vi "Write Frame Data Recorder Multi Tool.vi"(8 "error in (no error)":errorcluster, 9 "Append":bool, 10 "Rigid Bodies":T1[](array[typedef]), 11 "Frame Grabber Data In in":T5={"Camera Session"="", "Frame"=refnum, "AVI Refnum"=refnum, "Codecs"=[], "Frame number"=0, "Tracking File Refnum"=refnum, "Tick Count"=0, "Probe Object"=refnum, "Playback Probe Data"=[], "Rigid Body"={"Position"={"x (mm)"=0.0, "y (mm)"=0.0, "z (mm)"=0.0}, "Orientation"={"Pitch (rad)"=0.0, "Yaw (rad)"=0.0, "Roll (rad)"=0.0}, "Quaternion"={"qx"=0.0, "qy"=0.0, "qz"=0.0, "qw"=0.0}, "Tracked?"=FALSE}, "Total no frames playback"=0, "Video FPS"=0.0, "Camera connected?"=FALSE, "Scene"=refnum, "Cropped Frame"=refnum, "Tracker FPS"=0.0, "Crop ROI"=[], "Presentation Values"=[], "Elapsed time (ms)"=0, "Camera frames playback"=0, "Refnums"={"Live Refnum"=refnum, "Record Refnum"=refnum, "Playback Refnum"=refnum, "Frame Slider Refnum"=refnum, "Pause Refnum"=refnum, "Home Refnum"=refnum, "Set Crop Refnum"=refnum, "Clear Crop Refnum"=refnum, "stop refnum"=refnum, "Playback Rate Refnum"=refnum, "Presentation Refnum"=refnum, "Crop Time Frame Slider Refnum"=refnum, "Cancel Save Refnum"=refnum, "Reverse Playback Refnum"=refnum, "Recording Settings Refnum"=refnum, "Continuous Playback Refnum"=refnum, "Annotation Refnum"=refnum, "Export All Refnum"=refnum, "Export List Refnum"=refnum, "Fill List Refnum"=refnum, "Save Crop Refnum"=refnum, "Skip Forward Refnum"=refnum, "Skip Backward Refnum"=refnum, "Single Annotation Refnum"=refnum, "Load Video Refnum"=refnum, "Set Start Refnum"=refnum, "Set End Refnum"=refnum, "Add to List Refnum"=refnum, "List of Annotations Refnum"=refnum, "Camera Frame Refnum"=refnum, "Load Image Refnum"=refnum, "Saving Refnum"=refnum}, "Dimensions"={"Probe Dimensions"={"Probe Width"=0.0, "Probe Depth"=1.0, "Probe Height"=0.0}, "Room Dimensions"={"Room Width"=0.0, "Room Depth"=0.0, "Room Height"=0.0}}, "Playback Data As Strings"=[], "Cropped Tracking File Refnum"=refnum, "Cropped AVI Refnum"=refnum, "Header"=[], "Total euclidian distance"=0.0, "Annotation File Path"=path "", "Playback File Path"=path "", "Size per frame"=0.0, "Ground Truth File Refnum"=refnum, "Annotation Array"=[], "Annotation TIFFs Folder"=path "", "overwriting open file?"=FALSE, "Image Sequence"=[], "Video/Image Flag"=enum."Playback Video Frame", "Image sequence?"=FALSE, "Image sequence filenames"=[], "Mask"=refnum, "Crop Type"=enum."Rectangle"}) -> (0 "error out":errorcluster, 1 "Time elapsed (s)":dbl, 2 "Image":T4, 3 "Frame Grabber Data out":T5={"Camera Session"="", "Frame"=refnum, "AVI Refnum"=refnum, "Codecs"=[], "Frame number"=0, "Tracking File Refnum"=refnum, "Tick Count"=0, "Probe Object"=refnum, "Playback Probe Data"=[], "Rigid Body"={"Position"={"x (mm)"=0.0, "y (mm)"=0.0, "z (mm)"=0.0}, "Orientation"={"Pitch (rad)"=0.0, "Yaw (rad)"=0.0, "Roll (rad)"=0.0}, "Quaternion"={"qx"=0.0, "qy"=0.0, "qz"=0.0, "qw"=0.0}, "Tracked?"=FALSE}, "Total no frames playback"=0, "Video FPS"=0.0, "Camera connected?"=FALSE, "Scene"=refnum, "Cropped Frame"=refnum, "Tracker FPS"=0.0, "Crop ROI"=[], "Presentation Values"=[], "Elapsed time (ms)"=0, "Camera frames playback"=0, "Refnums"={"Live Refnum"=refnum, "Record Refnum"=refnum, "Playback Refnum"=refnum, "Frame Slider Refnum"=refnum, "Pause Refnum"=refnum, "Home Refnum"=refnum, "Set Crop Refnum"=refnum, "Clear Crop Refnum"=refnum, "stop refnum"=refnum, "Playback Rate Refnum"=refnum, "Presentation Refnum"=refnum, "Crop Time Frame Slider Refnum"=refnum, "Cancel Save Refnum"=refnum, "Reverse Playback Refnum"=refnum, "Recording Settings Refnum"=refnum, "Continuous Playback Refnum"=refnum, "Annotation Refnum"=refnum, "Export All Refnum"=refnum, "Export List Refnum"=refnum, "Fill List Refnum"=refnum, "Save Crop Refnum"=refnum, "Skip Forward Refnum"=refnum, "Skip Backward Refnum"=refnum, "Single Annotation Refnum"=refnum, "Load Video Refnum"=refnum, "Set Start Refnum"=refnum, "Set End Refnum"=refnum, "Add to List Refnum"=refnum, "List of Annotations Refnum"=refnum, "Camera Frame Refnum"=refnum, "Load Image Refnum"=refnum, "Saving Refnum"=refnum}, "Dimensions"={"Probe Dimensions"={"Probe Width"=0.0, "Probe Depth"=1.0, "Probe Height"=0.0}, "Room Dimensions"={"Room Width"=0.0, "Room Depth"=0.0, "Room Height"=0.0}}, "Playback Data As Strings"=[], "Cropped Tracking File Refnum"=refnum, "Cropped AVI Refnum"=refnum, "Header"=[], "Total euclidian distance"=0.0, "Annotation File Path"=path "", "Playback File Path"=path "", "Size per frame"=0.0, "Ground Truth File Refnum"=refnum, "Annotation Array"=[], "Annotation TIFFs Folder"=path "", "overwriting open file?"=FALSE, "Image Sequence"=[], "Video/Image Flag"=enum."Playback Video Frame", "Image sequence?"=FALSE, "Image sequence filenames"=[], "Mask"=refnum, "Crop Type"=enum."Rectangle"}, 4 "File Size (MB)":dbl, 5 "Greater than 2 GB?":bool)   [LabVIEW 2017]
uses:
  Controls/Frame Grabber Data.ctl
  <vilib>/userdefined/High Color/IMAQdx.ctl
  <vilib>/vision/Image Controls.llb/IMAQ Image.ctl
  <vilib>/vision/Avi.llb/IMAQ AVI2 Refnum.ctl
  Controls/Rigid Body Info.ctl
  Controls/Position.ctl
  Controls/Orientation.ctl
  Controls/Refnums.ctl
  Controls/Recording Settings.ctl
  Controls/Operator Settings.ctl
  Controls/Operator.ctl
  Controls/Patient Settings.ctl
  Controls/Dimensions.ctl
  Controls/Room Dimensions.ctl
  Controls/Crop Video State.ctl
  Controls/Crop Type.ctl
panel:
  out "Camera frame number":dbl
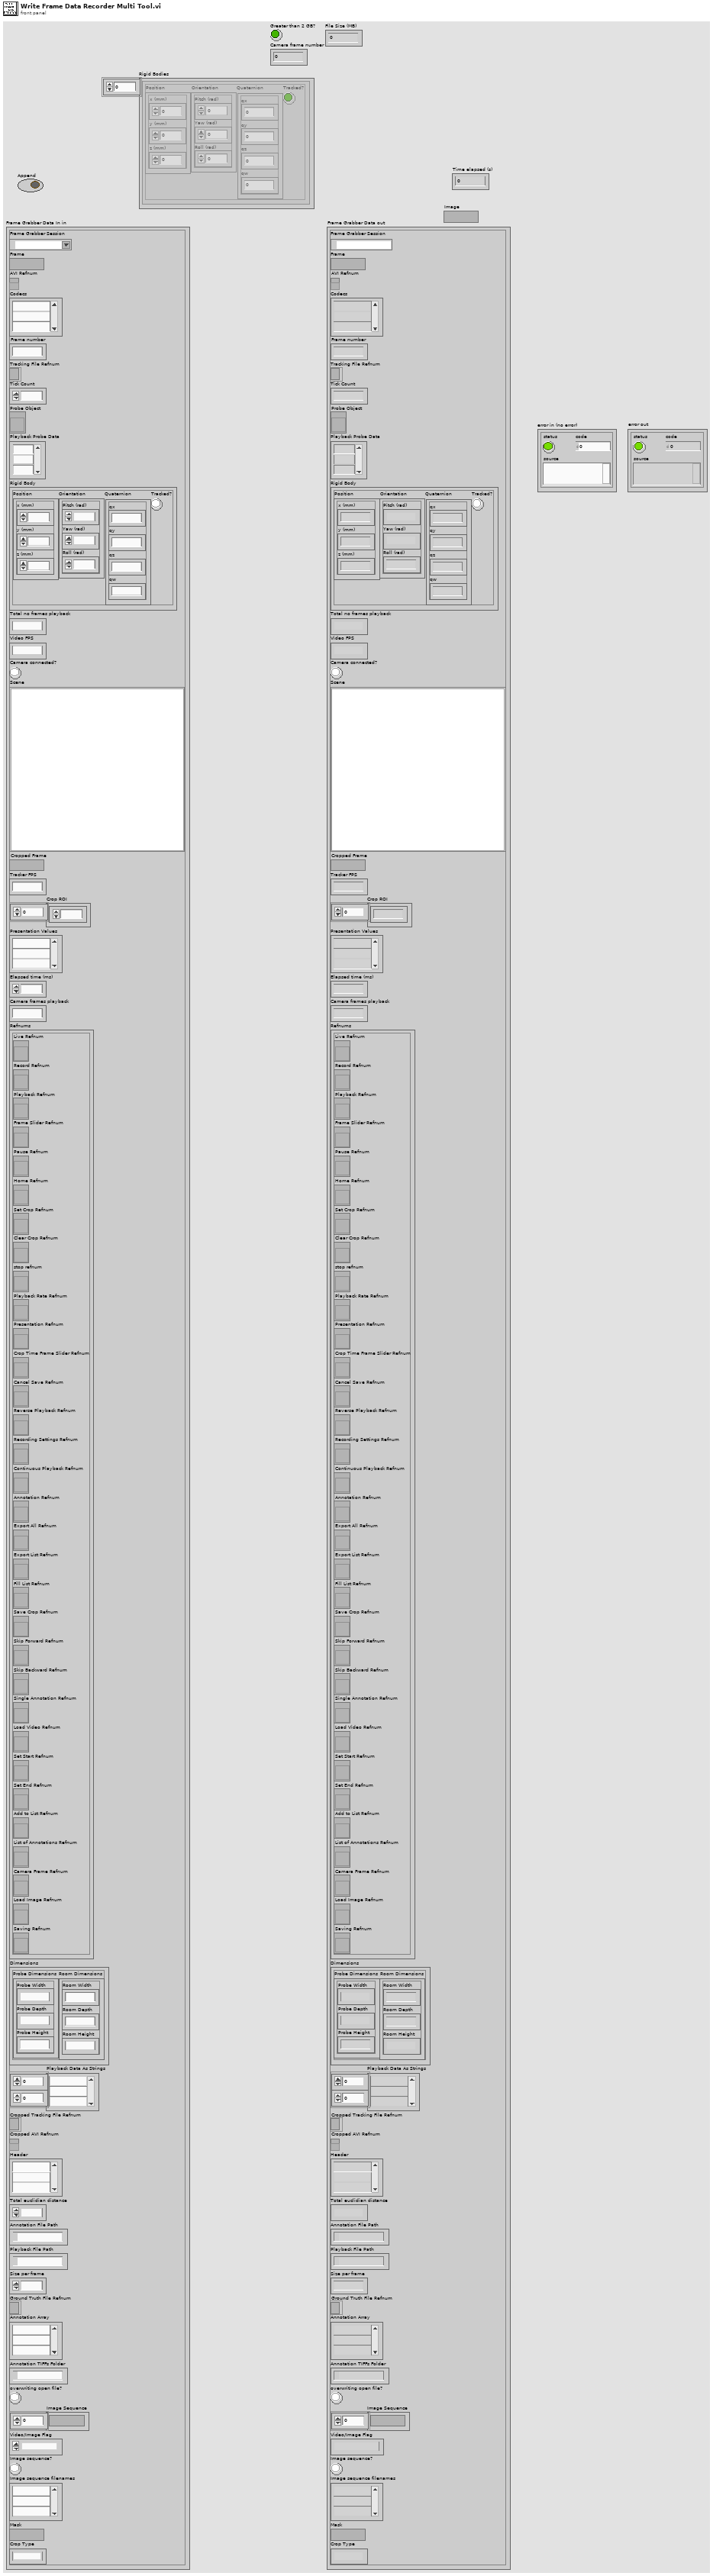
[diagram p1: front panel]
types:
  T1 = typedef "Rigid Body Info.ctl" = cluster{"Position":T2, "Orientation":T3, "Quaternion":cluster{"qx":sgl, "qy":sgl, "qz":sgl, "qw":sgl}, "Tracked?":bool}
  T2 = typedef "Position.ctl" = cluster{"x (mm)":sgl, "y (mm)":sgl, "z (mm)":sgl}
  T3 = typedef "Orientation.ctl" = cluster{"Pitch (rad)":sgl, "Yaw (rad)":sgl, "Roll (rad)":sgl}
  T4 = typedef "IMAQ Image.ctl" = refnum<image>
  T5 = typedef "Frame Grabber Data.ctl" = cluster{"Camera Session":T6, "Frame":T4, "AVI Refnum":T7, "Codecs":string[], "Frame number":u32, "Tracking File Refnum":refnum<file>, "Tick Count":u32, "Probe Object":refnum<vi>, "Playback Probe Data":dbl[][], "Rigid Body":T1, "Total no frames playback":i32, "Video FPS":dbl, "Camera connected?":bool, "Scene":refnum<vi>, "Cropped Frame":T4, "Tracker FPS":dbl, "Crop ROI":i32[], "Presentation Values":string[], "Elapsed time (ms)":u32, "Camera frames playback":u32, "Refnums":T8, "Dimensions":T9, "Playback Data As Strings":string[][], "Cropped Tracking File Refnum":refnum<file>, "Cropped AVI Refnum":T7, "Header":string[], "Total euclidian distance":dbl, "Annotation File Path":path, "Playback File Path":path, "Size per frame":dbl, "Ground Truth File Refnum":refnum<file>, "Annotation Array":string[], "Annotation TIFFs Folder":path, "overwriting open file?":bool, "Image Sequence":T4[], "Video/Image Flag":T11, "Image sequence?":bool, "Image sequence filenames":string[], "Mask":T4, "Crop Type":T12}
  T6 = typedef "IMAQdx.ctl" = refnum<k21>
  T7 = typedef "IMAQ AVI2 Refnum.ctl" = refnum<k20>
  T8 = typedef "Refnums.ctl" = cluster{"Live Refnum":refnum<vi>, "Record Refnum":refnum<vi>, "Playback Refnum":refnum<vi>, "Frame Slider Refnum":refnum<vi>, "Pause Refnum":refnum<vi>, "Home Refnum":refnum<vi>, "Set Crop Refnum":refnum<vi>, "Clear Crop Refnum":refnum<vi>, "stop refnum":refnum<vi>, "Playback Rate Refnum":refnum<vi>, "Presentation Refnum":refnum<vi>, "Crop Time Frame Slider Refnum":refnum<vi>, "Cancel Save Refnum":refnum<vi>, "Reverse Playback Refnum":refnum<vi>, "Recording Settings Refnum":refnum<vi>, "Continuous Playback Refnum":refnum<vi>, "Annotation Refnum":refnum<vi>, "Export All Refnum":refnum<vi>, "Export List Refnum":refnum<vi>, "Fill List Refnum":refnum<vi>, "Save Crop Refnum":refnum<vi>, "Skip Forward Refnum":refnum<vi>, "Skip Backward Refnum":refnum<vi>, "Single Annotation Refnum":refnum<vi>, "Load Video Refnum":refnum<vi>, "Set Start Refnum":refnum<vi>, "Set End Refnum":refnum<vi>, "Add to List Refnum":refnum<vi>, "List of Annotations Refnum":refnum<vi>, "Camera Frame Refnum":refnum<vi>, "Load Image Refnum":refnum<vi>, "Saving Refnum":refnum<vi>}
  T9 = typedef "Dimensions.ctl" = cluster{"Probe Dimensions":cluster{"Probe Width":sgl, "Probe Depth":sgl, "Probe Height":sgl}, "Room Dimensions":T10}
  T10 = typedef "Room Dimensions.ctl" = cluster{"Room Width":dbl, "Room Depth":dbl, "Room Height":dbl}
  T11 = typedef "Crop Video State.ctl" = enum16{"Init", "Wait", "Load Image", "Load Video", "Play/Pause", "Playback Video Frame", "Display Image", "Save Image Sequence", "Save Video", "Export List", "Export All", "Close", "Set Crop Area", "Reset Crop Area", "Crop Inside", "Crop Outside", "Multi-Crop", "Re-Open Files", "Annotate Frame", "Annotate Clip", "Add to List", "Fill List", "Set Start", "Set End", "Error Handling", "Shutdown"}
  T12 = typedef "Crop Type.ctl" = enum16{"Rectangle", "Annulus"}
  T13 = typedef "Recording Settings.ctl" = cluster{"Folder to Save Recordings":path, "Video FPS":u32, "Codec":u16, "Tracker FPS":u32, "Operator ID":T14, "Patient ID/Gestation":T16}
  T14 = typedef "Operator Settings.ctl" = cluster{"Operator ID":u32, "Expertise":T15}
  T15 = typedef "Operator.ctl" = u16
  T16 = typedef "Patient Settings.ctl" = cluster{"ID":u32, "Gestation":string}
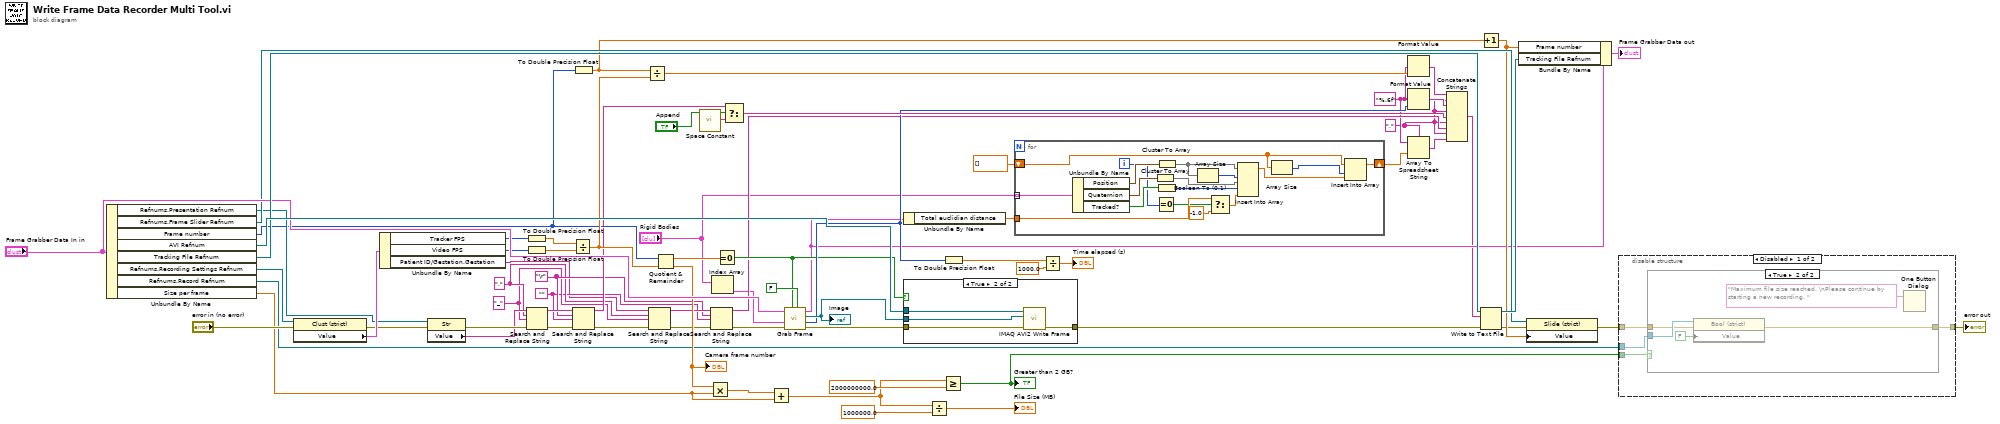
[diagram p0: block diagram]
diagram:
  w3 = "," ("delimiter (Tab)")
  w5 = "%.6f" ("format string")
  w20 = ""
  w23 = "\r"
  w21 = "_" ("replace string (\"\")")
  w22 = "," ("search string")
  n1 = Unbundle By Name("Frame Grabber Data In in") -> ("Refnums.Presentation Refnum"=w47:refnum<vi>, "Refnums.Frame Slider Refnum"=w64:refnum<vi>, "Frame number"=w43:u32, "AVI Refnum"=w71:T7, "Tracking File Refnum"=w70:refnum<file>, "Refnums.Recording Settings Refnum"=w50:refnum<vi>, "Refnums.Record Refnum"=w34:refnum<vi>, "Size per frame"=w16:dbl)
  n2 = property class="Clust (strict)"(reference=w50, error in="error in (no error)") -> (error out=w46:errorcluster, "Value"=w49:T13)  [unwired: 1 out]
  n3 = Unbundle By Name(w49) -> ("Tracker FPS"=w61:u32, "Video FPS"=w58:u32, "Patient ID/Gestation.Gestation"=w15:string)
  n4 = property class="Str"(reference=w47, error in=w46) -> (error out=w33:errorcluster, "Value"=w32:string)  [unwired: 1 out]
  n5 = To Double Precision Float(number=w61) -> (double precision float=w14:dbl)
  n6 = To Double Precision Float(number=w58) -> (double precision float=w13:dbl)
  n7 = Search and Replace String(input string=w32, search string=w22, replace string=w21, error in=w33) -> (result string=w29:string, error out=w31:errorcluster)  [unwired: 4 in, 2 out]
  n8 = Divide(x=w14, y=w13) -> (x/y=w55:dbl)
  n9 = Search and Replace String(input string=w29, search string=w23, replace string=w20, error in=w31) -> (result string=w28:string, error out=w30:errorcluster)  [unwired: 4 in, 2 out]
  n10 = To Double Precision Float(number=w43) -> (double precision float=w45:dbl)
  n11 = Divide(x=w45, y=w55) -> (x/y=w44:dbl)
  n12 = Search and Replace String(input string=w15, search string=w22, replace string=w21, error in=w30) -> (result string=w26:string, error out=w27:errorcluster)  [unwired: 4 in, 2 out]
  n13 = Quotient & Remainder(x=w43, y=w55) -> (x-y*floor(x/y)=w59:dbl, floor(x/y)=w41:dbl)
  "Camera frame number" <- w41
  n14 = call <vilib>:"Space Constant.vi"() -> ("String"=w62:string)
  n15 = Multiply(x=w41, y=w16) -> (x*y=w40:dbl)
  n16 = Search and Replace String(input string=w26, search string=w23, replace string=w20, error in=w27) -> (result string=w25:string, error out=w24:errorcluster)  [unwired: 4 in, 2 out]
  n17 = Index Array(array="Rigid Bodies") -> (element=w12:T1)  [unwired: 1 in]
  n18 = Equal To 0?(x=w59) -> (x = 0?=w42:bool)
  n19 = Select(t=w28, s="Append", f=w62) -> (s? t:f=w56:string)
  n20 = Add(x=w40, y=w16) -> (x+y=w38:dbl)
  n21 = call "Grab Frame.vi"("Live?"=FALSE, "Grab frame?"=w42, "error in (no error)"=w24, "Rigid Body"=w12, "Frame Grabber Data in"="Frame Grabber Data In in") -> ("error out"=w67:errorcluster, "Elapsed time (ms)"=w54:u32, "Frame"=w68:T4, "Frame Grabber Data out"=w19:T5)  [unwired: 3 in]
  "Image" <- w68
  n22 = Unbundle By Name(w19) -> ("Total euclidian distance"=w6:dbl)
  n23 = case shown="True" w42 {
    tunnel: [w73 w77] -> w72
    tunnel: w71 -> [_ w76]
    tunnel: w68 -> [_ w75]
    tunnel: w67 -> [w73 w74]
    frame False {
    }
    frame True {
      n24 = call "IMAQ AVI2 Write Frame"("error in (no error)"=w74, "Image"=w75, "AVI Refnum"=w76) -> ("error out"=w77:errorcluster)  [unwired: 6 in, 2 out]
    }
  }
  n25 = Divide(x=w38, y=1000000.0) -> (x/y=→"File Size (MB)":dbl)
  n26 = Greater Or Equal?(x=w38, y=2000000000.0) -> (x >= y?=w37:bool)
  "Greater than 2 GB?" <- w37
  n27 = To Double Precision Float(number=w54) -> (double precision float=w52:dbl)
  n28 = for {
    tunnel: "Rigid Bodies" -> [w94] mode=indexing
    tunnel: w6 -> [w93]
    shift-right: [w82] -> w4
    shift-left: sgl[] [] -> [w79]
    i -> [w81]
    n29 = Unbundle By Name(w94) -> ("Position"=w88:T2, "Quaternion"=w92:cluster{"qx":sgl, "qy":sgl, "qz":sgl, "qw":sgl}, "Tracked?"=w87:bool)
    n30 = Cluster To Array(cluster=w92) -> (array=w89:sgl[])
    n31 = Boolean To (0,1)(Boolean=w87) -> (0, 1=w86:i16)
    n32 = Equal To 0?(x=w81) -> (x = 0?=w85:bool)
    n33 = Cluster To Array(cluster=w88) -> (array=w90:sgl[])
    n34 = Array Size(array=w90) -> (size(s)=w91:i32)
    n35 = Select(t=w93, s=w85, f=-1.0) -> (s? t:f=w83:dbl)
    n36 = Insert Into Array(array=w90, index=w91, new element #1=w89, new element #2=w86, new element #3=w83) -> (w80:sgl[])
    n37 = Array Size(array=w79) -> (size(s)=w78:i32)
    n38 = Insert Into Array(array=w79, index=w78, new element=w80) -> (w82:sgl[])
  }
  n39 = Divide(x=w52, y=1000.0) -> (x/y=→"Time elapsed (s)":dbl)
  n40 = Format Value(format string=w5, value (0)=w44) -> (output string=w8:string)  [unwired: 1 in]
  n41 = Format Value(format string=w5, value (0)=w54) -> (output string=w7:string)  [unwired: 1 in]
  n42 = Array To Spreadsheet String(delimiter (Tab)=w3, array=w4, 3:w5) -> (spreadsheet string=w2:string)
  n43 = Concatenate Strings(w8, w3, w7, w3, w56, w3, w25, w3, w2) -> (w9:string)
  n44 = Increment(x=w45) -> (x+1=w63:dbl)
  n45 = Write to Text File(file (use dialog)=w70, text=w9, error in=w72) -> (refnum out=w69:refnum<file>, error out=w10:errorcluster)  [unwired: 1 in, 1 out]
  n46 = Bundle By Name(cluster=w19, "Frame number"=w63, "Tracking File Refnum"=w69) -> (→"Frame Grabber Data out":T5)
  n47 = property class="Slide (strict)"(reference=w64, error in=w10, "Value"=w63) -> (error out=w36:errorcluster)  [unwired: 1 out]
  n48 = disable-structure shown="Disabled" {
    disable-tunnel: w37 -> [w98 _]
    disable-tunnel: w36 -> [w97 w105]
    disable-tunnel: [w96 w105] -> w35
    disable-tunnel: w34 -> [w95 _]
    frame Disabled {
      n49 = case shown="True" w98 {
        tunnel: w97 -> [w99 w102]
        tunnel: [w99 w101] -> w96
        tunnel: w95 -> [_ w103]
        frame False {
        }
        frame True {
          n50 = property class="Bool (strict)"(reference=w103, error in=w102, "Value"=FALSE) -> (error out=w101:errorcluster)  [unwired: 1 out]
          n51 = One Button Dialog(message="Maximum file size reached. \nPlease continue by starting a new recording. ") -> ()  [unwired: 1 in, 1 out]
        }
      }
    }
    frame Enabled {
    }
  }
  "error out" <- w35
